vi "Example.vi"() -> ()   [LabVIEW 2018]
uses:
  Data Def/Mitsubishi_Batch Read In Word Units Command.ctl
  Data Def/Mitsubishi_Device Code.ctl
  Data Def/Mitsubishi_Registers Data Type.ctl
  Data Def/Mitsubishi_Read Response Message.ctl
  Data Def/Mitsubishi_Request Type.ctl
  Data Def/Mitsubishi_Batch Write In Word Units Command.ctl
  Data Def/Mitsubishi_Request Message Format.ctl
  Data Def/Mitsubishi_Access Route.ctl
panel:
  in  "Message Format":T1={"Access Route"={"Network No."="\u0000", "PC No."="ÿ", "Module I/O No."="\u0003", "Module Station No."="\u0000"}, "Monitoring Timer(ms)"=4000, "Request Type"=enum."Batch read in word units", "Request Data"=variant}
  out "error out":errorcluster
  in  "Request Type":T3
  out "Response Message":T4 {"Subheader" format="%.0x"; "Access Route"."Network No." format="%.0x"; "Access Route"."PC No." format="%.0x"; "Access Route"."Module I/O No." format="%.0x"; "Access Route"."Module Station No." format="%.0x"; "End Code" format="%.0x"; "Response Data" format="%.0x"}
  out "Request Message":string
  in  "Tab Control":enum32{"Batch Read", "Batch Write"}(tab)
  in  "Batch Read In Word Units":T5={"Head Device Number"=0, "Device Code"=168, "Number Of Device Point"=700, "Registers Data Type"=enum."16 Bit int"} {"Device Code" items=["SM"=145, "SD"=169, "X*"=156, "Y*"=157, "M*"=144, "L*"=146, "F*"=147, "V*"=148, "B*"=160, "D*"=168, "W*"=180, "TS"=193, "TC"=192, "TN"=194, "SS"=199, "SC"=198, "SN"=200, "CS"=196, "CC"=195, "CN"=197, "SB"=161, "SW"=181, "S*"=152, "DX"=162, "DY"=163, "Z*"=204, "R*"=175, "ZR"=176, "G"=171]}
  out "Response Data":i16[](array[numeric])
  out "Boolean array":bool[][](array[boolean])
  in  "Batch Write In Word Units":T8={"Head Device Number"=0, "Device Code"=168, "Write Data"=[]} {"Write Data" format="%.0x"; "Device Code" items=["SM"=145, "SD"=169, "X*"=156, "Y*"=157, "M*"=144, "L*"=146, "F*"=147, "V*"=148, "B*"=160, "D*"=168, "W*"=180, "TS"=193, "TC"=192, "TN"=194, "SS"=199, "SC"=198, "SN"=200, "CS"=196, "CC"=195, "CN"=197, "SB"=161, "SW"=181, "S*"=152, "DX"=162, "DY"=163, "Z*"=204, "R*"=175, "ZR"=176, "G"=171]}
  out "Time":u32
  in  "stop":bool
  out "Respond Data":string
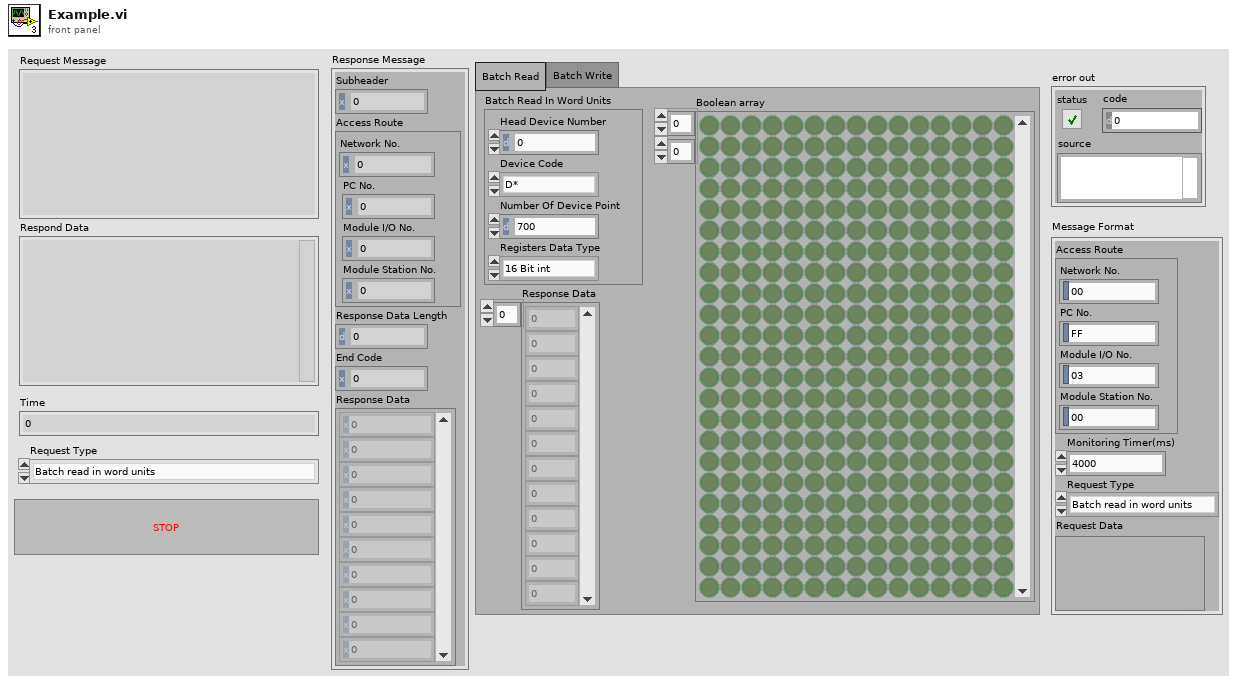
[diagram p1: front panel]
types:
  T1 = typedef "Mitsubishi_Request Message Format.ctl" = cluster{"Access Route":T2, "Monitoring Timer(ms)":u16, "Request Type":T3, "Request Data":variant}
  T2 = typedef "Mitsubishi_Access Route.ctl" = cluster{"Network No.":string, "PC No.":string, "Module I/O No.":string, "Module Station No.":string}
  T3 = typedef "Mitsubishi_Request Type.ctl" = enum16{"Batch read in word units", "Batch write in word units"}
  T4 = typedef "Mitsubishi_Read Response Message.ctl" = cluster{"Subheader":u16, "Access Route":cluster{"Network No.":u8, "PC No.":u8, "Module I/O No.":u16, "Module Station No.":u8}, "Response Data Length":u8, "End Code":u16, "Response Data":i16[]}
  T5 = typedef "Mitsubishi_Batch Read In Word Units Command.ctl" = cluster{"Head Device Number":u16, "Device Code":T6, "Number Of Device Point":u16, "Registers Data Type":T7}
  T6 = typedef "Mitsubishi_Device Code.ctl" = u8
  T7 = typedef "Mitsubishi_Registers Data Type.ctl" = enum16{"16 Bit int", "16 Bit Uint", "32 Bit int", "32 Bit Uint", "32 Bit float", "64 Bit double", "Characters"}
  T8 = typedef "Mitsubishi_Batch Write In Word Units Command.ctl" = cluster{"Head Device Number":u16, "Device Code":T6, "Write Data":i16[]}
  T9 = enum16{"Standard", "Buffered", "CRLF", "Immediate"}
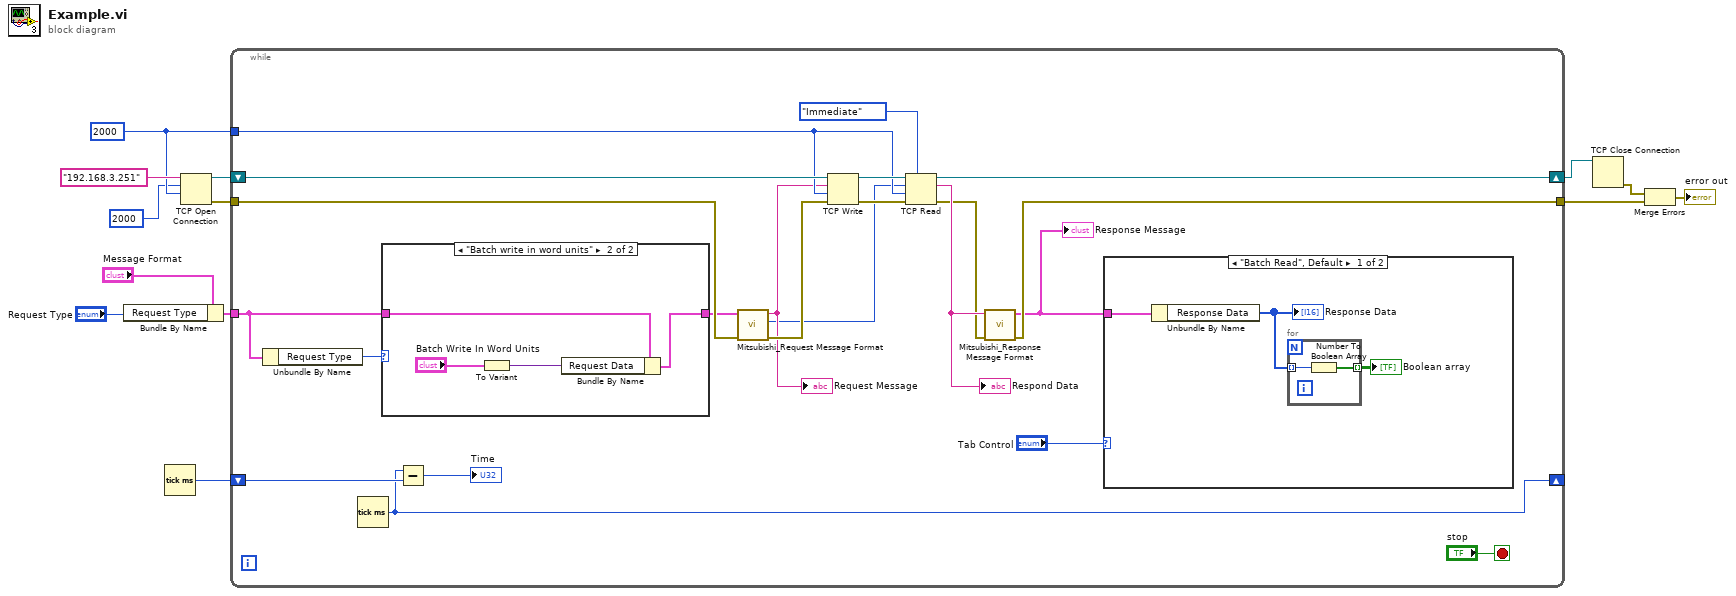
[diagram p0: block diagram]
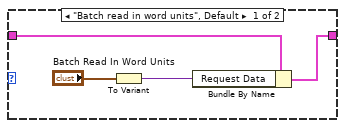
[diagram p3: hidden frame]
diagram:
  w10 = 2000 ("timeout ms (60000)")
  n1 = Bundle By Name(cluster="Message Format", "Request Type"="Request Type") -> (w6:T1)
  n2 = Tick Count (ms)() -> (millisecond timer value=w9:u32)
  n3 = TCP Open Connection(address="192.168.3.251", remote port or service name=u16 2000, timeout ms (60000)=w10) -> (connection ID=w11:refnum<k5>, error out=w12:errorcluster)  [unwired: 2 in]
  n4 = while {
    tunnel: w10 -> [w32]
    shift-right: [w33] -> w4
    shift-left: w11 -> [w35]
    shift-right: [w27] -> _
    shift-left: w9 -> [w28]
    tunnel: w6 -> [w20]
    tunnel: w12 -> [w25]
    tunnel: [w16] -> w3
    stop <- "stop" stop-if-true
    n5 = Unbundle By Name(w20) -> ("Request Type"=w21:T3)
    n6 = Tick Count (ms)() -> (millisecond timer value=w27:u32)
    n7 = case shown="\"Batch write in word units\"" w21 {
      tunnel: w20 -> [w44 w48]
      tunnel: [w41 w45] -> w19
      frame "Batch read in word units", Default {
        n8 = To Variant(anything="Batch Read In Word Units") -> (Variant=w42:variant)
        n9 = Bundle By Name(cluster=w44, "Request Data"=w42) -> (w41:T1)
      }
      frame "Batch write in word units" {
        n10 = To Variant(anything="Batch Write In Word Units") -> (Variant=w46:variant)
        n11 = Bundle By Name(cluster=w48, "Request Data"=w46) -> (w45:T1)
      }
    }
    n12 = Subtract(x=w27, y=w28) -> (x-y=→"Time":u32)
    n13 = call "Mitsubishi_Request Message Format.vi"("error in"=w25, "Request Message Format"=w19) -> ("error out"=w24:errorcluster, "Byte To Read"=w22:i32, "Request Message"=w23:string)  [unwired: 7 in]
    "Request Message" <- w23
    n14 = TCP Write(connection ID=w35, data in=w23, error in (no error)=w24, 9:w32) -> (connection ID out=w34:refnum<k5>, error out=w29:errorcluster)  [unwired: 1 out]
    n15 = TCP Read(connection ID=w34, bytes to read=w22, error in (no error)=w29, 7:T9."Immediate" ("mode (standard)"), 9:w32) -> (connection ID out=w33:refnum<k5>, data out=w18:string, error out=w17:errorcluster)
    "Respond Data" <- w18
    n16 = call "Mitsubishi_Response Message Format.vi"("error in"=w17, "Respond Data"=w18) -> ("error out"=w16:errorcluster, "Response Message"=w15:T4)  [unwired: 8 in]
    "Response Message" <- w15
    n17 = case shown="\"Batch Read\", Default" "Tab Control" {
      tunnel: w15 -> [w38 _]
      frame "Batch Read", Default {
        n18 = Unbundle By Name(w38) -> ("Response Data"=w36:i16[])
        "Response Data" <- w36
        n19 = for {
          tunnel: w36 -> [w40] mode=indexing
          tunnel: [w39] -> w37 mode=indexing
          n20 = Number To Boolean Array(number=w40) -> (Boolean array=w39:bool[])
        }
        "Boolean array" <- w37
      }
      frame "Batch Write" {
      }
    }
  }
  n21 = TCP Close Connection(connection ID=w4) -> (error out=w2:errorcluster)  [unwired: 2 in, 1 out]
  n22 = Merge Errors(w2, w3) -> (→"error out":errorcluster)
